vi "Out_S2F13.vi"(8 "error in (no error)":errorcluster, 11 "S2 Message Class in":refnum<class "S2 Message Class.lvclass">) -> (0 "error out":errorcluster, 3 "S2 Message Class out":refnum<class "S2 Message Class.lvclass">)   [LabVIEW 2020, in "SECS Communication.lvlib" / "S2 Message Class.lvclass"]
uses:
  S2 Message Class.lvclass
  D:/Dropbox/SECS/SECS_GEM v1.0.6/Com/SECS Communication/SECS-II Class/SECS-II Class.lvclass
  SECS-II Class/Data Message_List.vi
  SECS-II Class/Data Message_U4.vi
  SECS-II Class/SECS-II Class.lvclass
  D:/Dropbox/SECS/SECS_GEM v1.0.6/Com/SECS Communication/S2 Message Class/S2 Message Class.lvclass
panel:
  in  "Equipment Constant ID(ECID)":u32[](array[numeric])
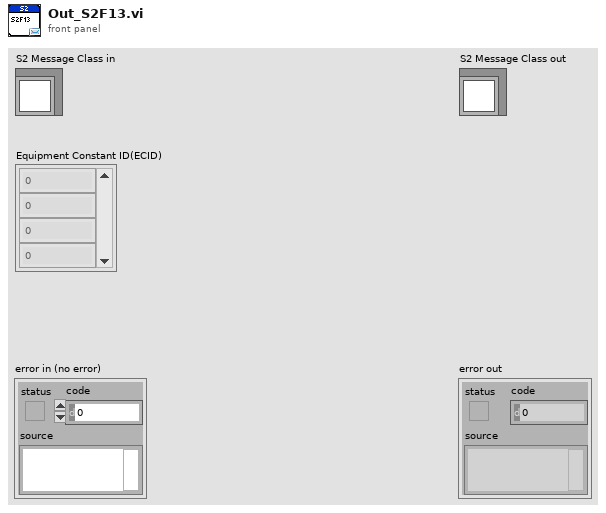
[diagram p1: front panel]
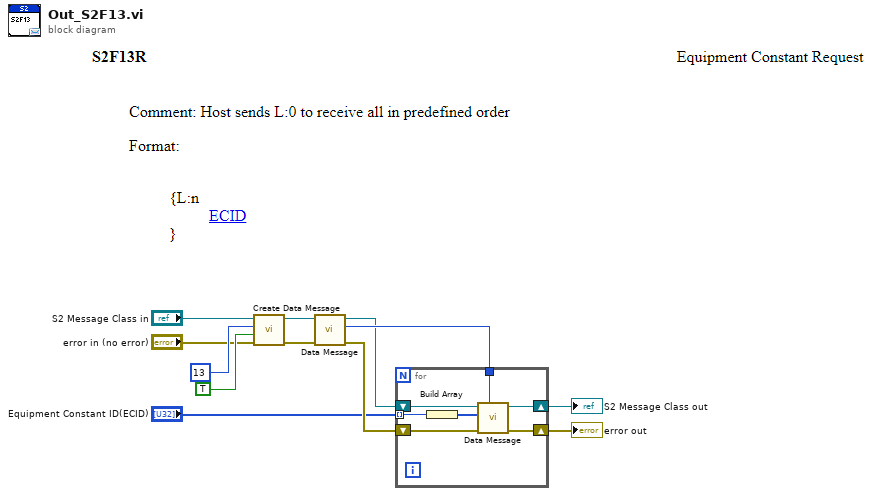
[diagram p0: block diagram]
diagram:
  n1 = call "Create Data Message.vi"("error in (no error)"="error in (no error)", "W-Bit"=TRUE, "Function"=u8 13, "SECS-II Class in"="S2 Message Class in") -> ("error out"=w8:errorcluster, "SECS-II Class out"=w9:refnum<class "S2 Message Class.lvclass">)  [unwired: 6 in]
  n2 = call-poly "Data Message.vi"("error in"=w8, "SECS-II Class in"=w9) -> ("error out"=w7:errorcluster, "Index"=w10:i32, "SECS-II Class out"=w6:refnum<class "S2 Message Class.lvclass">)  [unwired: 7 in]
  n3 = for {
    tunnel: w10 -> [w18]
    tunnel: "Equipment Constant ID(ECID)" -> [w14] mode=indexing
    shift-right: [w19] -> w2
    shift-left: w7 -> [w17]
    shift-right: [w15] -> w3
    shift-left: w6 -> [w16]
    n4 = Build Array(w14) -> (w13:u32[])
    n5 = call-poly "Data Message.vi"("Parent Index"=w18, "error in"=w17, "Data"=w13, "SECS-II Class in"=w16) -> ("error out"=w19:errorcluster, "SECS-II Class out"=w15:refnum<class "S2 Message Class.lvclass">)  [unwired: 6 in]
  }
  "error out" <- w2
  "S2 Message Class out" <- w3
